vi "PRF_Off.vi"(10 "Location":T5, 11 "Motion Settings In":T1 {"3rd Axis" items=["x", "y", "z", "w"]; "Xtra planes" min=1; "Xtra plane\ndistance  (um)" min=0; "Distance between\nscan planes (um)" format="%.2f"; "Distance between\nscan lines (um)" format="%.2f"; "SMAC Axis" items=["None"=0, "Axis 1"=1, "Axis 2"=2, "Axis 3"=3, "Axis 4"=4, "Axis 5"=5, "Axis 6"=6, "Axis 7"=7, "Axis 8"=8, "Vector Space 1"=17, "Vector Space 2"=18, "Vector Space 3"=19, "Vector Space 4"=20]; "Motion Bd ID" min=1 max=32 step=1}) -> (3 "Motion Settings Out":T1 {"3rd Axis" items=["x", "y", "z", "w"]; "Xtra planes" min=1; "Xtra plane\ndistance  (um)" min=0; "Distance between\nscan planes (um)" format="%.2f"; "Distance between\nscan lines (um)" format="%.2f"; "SMAC Axis" items=["None"=0, "Axis 1"=1, "Axis 2"=2, "Axis 3"=3, "Axis 4"=4, "Axis 5"=5, "Axis 6"=6, "Axis 7"=7, "Axis 8"=8, "Vector Space 1"=17, "Vector Space 2"=18, "Vector Space 3"=19, "Vector Space 4"=20]; "Motion Bd ID" min=1 max=32 step=1})   [LabVIEW 2022 SP3]
uses:
  Motion Controllers/NI_controller/-NI_MotionRoutines/MotionParameters.ctl
  Motion Controllers/NI_controller/-NI_MotionRoutines/MotionSys.ctl
  Motion Controllers/-MotionRoutines/ScanAxis.ctl
  Motion Controllers/-MotionRoutines/3rdAxis.ctl
  Controls/location.ctl
  Motion Controllers/Galil/Command Menu.ctl
  <vilib>/Motion/FlexMotion/FunctionsVIs/MotionIO.llb/Set Breakpoint Output MOMO (6 axes).flx
  <instrlib>/Newport ESP301/Newport ESP301.lvlib
panel:
  # "1-D and 2-D B scan settings"
  # "1-D and 2-D B scan settings"
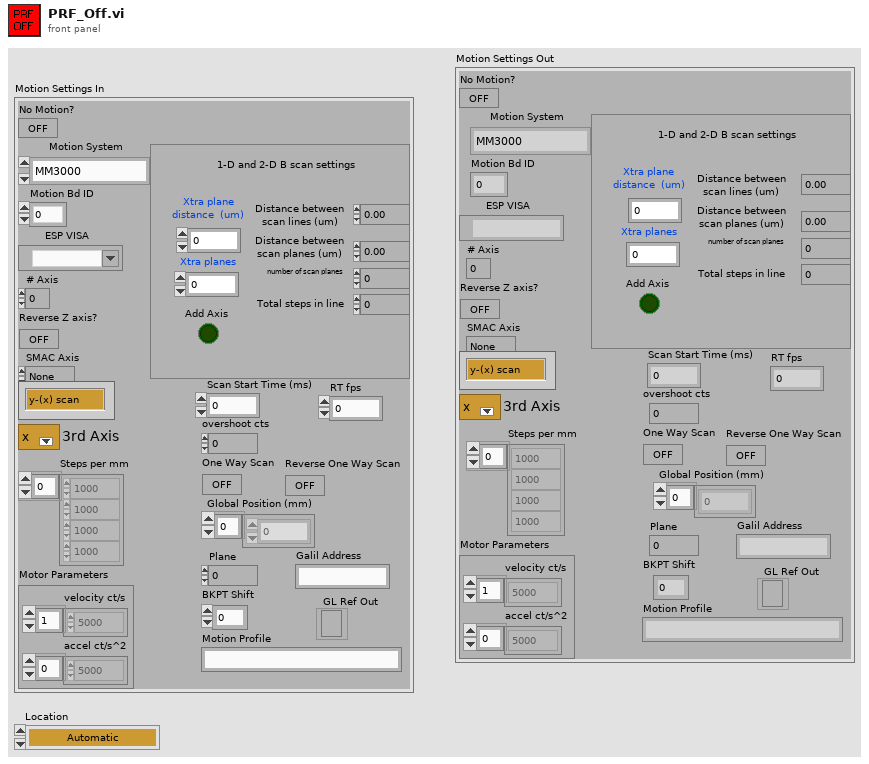
[diagram p1: front panel]
types:
  T1 = typedef "MotionParameters.ctl" = cluster{"No Motion?":bool, "Motion System":T2, "Motion Bd ID":u8, "Motion Profile":string, "# Axis":i8, "Reverse Z axis?":bool, "SMAC Axis":u16, "scan pair":T3, "RT fps":sgl, "Steps per mm":i32[], "Motor Parameters":cluster{"velocity ct/s":dbl[], "accel ct/s^2":dbl[]}, "One Way Scan":bool, "Reverse One Way Scan":bool, "Global Position (mm)":dbl[], "Plane":i32, "Distance between\nscan lines (um)":sgl, "Distance between\nscan planes (um)":sgl, "number of scan planes":i32, "Total steps in line":i32, "Xtra plane\ndistance  (um)":i32, "Xtra planes ":i32, "Add Axis":bool, "overshoot cts":i32, "BKPT Shift":i32, "Scan Start Time (ms)":u32, "ESP VISA":refnum<visa-resource-name>, "3rd Axis":T4, "GL Ref Out":refnum<k7>, "Galil Address":string}
  T2 = typedef "MotionSys.ctl" = enum16{"MM3000", "NI 735x", "Newport ESP", "No Motion Card", "Galil"}
  T3 = typedef "ScanAxis.ctl" = enum16{"y-(x) scan", "x-(y) scan", "z-(x) scan", "z-(y) scan", "y-(z) scan", "x-(z) scan", "w-(x) scan", "w-(y) scan", "w-(z) scan", "x-(w) scan", "y-(w) scan", "z-(w) scan"}
  T4 = typedef "3rdAxis.ctl" = u16
  T5 = typedef "location.ctl" = enum16{"Automatic", "WCM Main", "Hawaii", "Columbia MM3000", "Columbia  NI System", "NYU", "RRI 2", "UHI Allen", "CUMC RT", "Chiba", "Stony Brook", "WCM Microscopy", "WCM Aeoretch", "WCM Optics Lab", "WCM Main 2Axis", "WCM Rotation", "WCM SAM SMAC", "SERI GP"}
  T6 = cluster{"1":bool, "2":bool, "3":bool, "4":bool, "5":bool, "6":bool}
  T7 = typedef "Command Menu.ctl" = enum16{"CommandPassThrough", "Abort Motion", "Define Pos", "Velocity", "Acceleration", "Deceleration", "Position Rel", "Postion Abs", "Begin Move", "After Move", "Home", "KI", "KD", "KP", "IL", "Config I/O", "Set Bit", "Clear Bit", "Motor Off", "Moto On", "Status", "Execute", "Halt Execute", "HX Status", "Tell Velocity", "Check Motion", "BreakPoint", "Tell Position", "Current Code Line", "Tell Switches", "OC Force On", "OC Off", "Pos Soft Limit", "Rev Soft Limit"}
  T8 = typedef "Bd Id Out" = u8
  T9 = cluster{"Port A bit-0 at logic level":bool, "Port A bit-1 at logic level":bool, "Port A bit-2 at logic level ":bool, "Port A bit-3 at logic level":bool, "Port A bit-4 at logic level":bool, "Port A bit-5 at logic level ":bool, "Port A bit-6 at logic level ":bool, "Port A bit-7 at logic level ":bool, "Port B bit-0 at logic level":bool, "Port B bit-1 at logic level":bool, "Port B bit-2 at logic level ":bool, "Port B bit-3 at logic level":bool, "Port B bit-4 at logic level":bool, "Port B bit-5 at logic level ":bool, "Port B bit-6 at logic level ":bool, "Port B bit-7 at logic level ":bool}
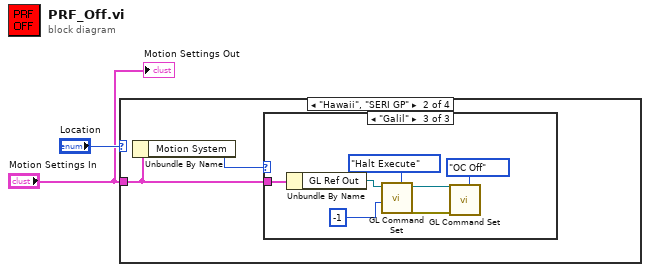
[diagram p0: block diagram]
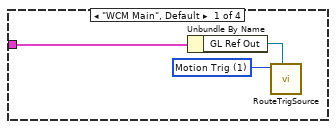
[diagram p2: hidden frame]
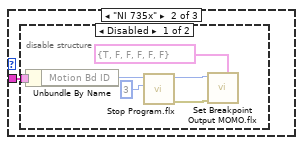
[diagram p4: hidden frame]
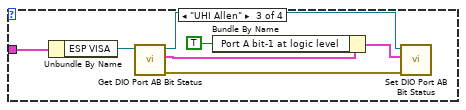
[diagram p6: hidden frame]
diagram:
  n1 = case shown="\"Hawaii\", \"SERI GP\"" "Location" {
    tunnel: "Motion Settings In" -> [w4 w7 w23 _]
    frame "WCM Main", Default {
      w5 = u16 1 items=["Function Gen Input", "Motion Trig", "Internal RT Motion Trig", "Internal CTR 1 Output"] ("Trig Source")
      n2 = Unbundle By Name(w4) -> ("GL Ref Out"=w3:refnum<k7>)
      n3 = call "RouteTrigSource.vi"("Galil.IGalil"=w3, "Trig Source"=w5) -> ()  [unwired: 9 in, 1 out]
    }
    frame "Hawaii", "SERI GP" {
      n4 = Unbundle By Name(w7) -> ("Motion System"=w6:T2)
      n5 = case shown="\"Galil\"" w6 {
        tunnel: w7 -> [_ w8 w21]
        frame "MM3000", Default {
        }
        frame "NI 735x" {
          n6 = disable-structure shown="Disabled" {
            disable-tunnel: w8 -> [w9 _]
            frame Disabled {
              n7 = Unbundle By Name(w9) -> ("Motion Bd ID"=w10:u8)
              n8 = call <vilib>:"Stop Program.flx"("Program (1)"=3, "Board ID"=w10) -> ("error out"=w11:errorcluster, "Bd ID Out"=w12:T8)  [unwired: 1 in, 4 out]
              n9 = call-poly <vilib>:"Set Breakpoint Output MOMO.flx"("Must Off"=T6 {"1"=TRUE, "2"=FALSE, "3"=FALSE, "4"=FALSE, "5"=FALSE, "6"=FALSE} ("Must On"), "error in (no error)"=w11, "Board ID"=w12) -> ()  [unwired: 3 in, 4 out]
            }
            frame Enabled {
            }
          }
        }
        frame "Galil" {
          n10 = Unbundle By Name(w21) -> ("GL Ref Out"=w20:refnum<k7>)
          n11 = call "GL Command Set.vi"("Command"=Command_Menu."Halt Execute", "Value"=-1, "Galil.IGalil"=w20) -> ("error out"=w18:errorcluster, "ref out"=w19:refnum<k7>)  [unwired: 4 in, 3 out]
          n12 = call "GL Command Set.vi"("Command"=Command_Menu."OC Off", "error in (no error)"=w18, "Galil.IGalil"=w19) -> ()  [unwired: 4 in, 5 out]
        }
      }
    }
    frame "UHI Allen" {
      n13 = Unbundle By Name(w23) -> ("ESP VISA"=w22:refnum<visa-resource-name>)
      n14 = call <instrlib>:"Get DIO Port AB Bit Status.vi"("VISA resource name"=w22) -> ("error out"=w25:errorcluster, "DIO Port A status"=w28:T9, "VISA resource name out"=w24:refnum<visa-resource-name>)  [unwired: 4 in]
      n15 = Bundle By Name(cluster=w28, "Port A bit-1 at logic level"=TRUE) -> (w26:T9)
      n16 = call <instrlib>:"Set DIO Port AB Bit Status.vi"("error in (no error)"=w25, "DIO Port status"=w26, "VISA resource name"=w24) -> ()  [unwired: 3 in, 2 out]
    }
    frame "CUMC RT" {
    }
  }
  "Motion Settings Out" <- "Motion Settings In"
